vi "Read Total A-Scans.vi"(8 "error in (no error)":errorcluster, 11 "Scan in":refnum<class "Scan.lvclass">) -> (0 "error out":errorcluster, 2 "Total A-Scans":dbl, 3 "Scan out":refnum<class "Scan.lvclass">)   [LabVIEW 2017]
uses:
  Scan.lvclass
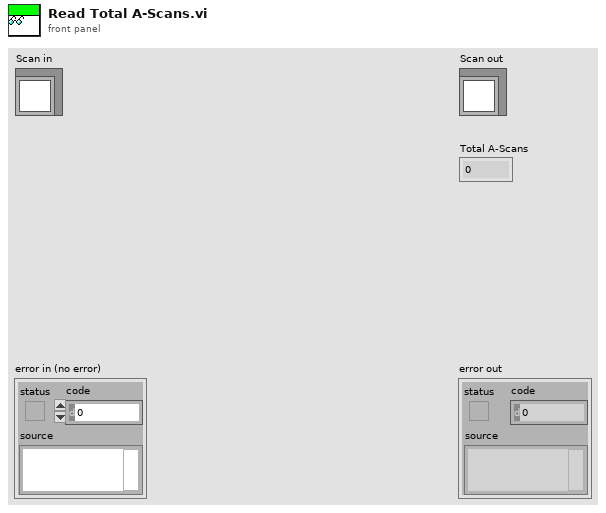
[diagram p1: front panel]
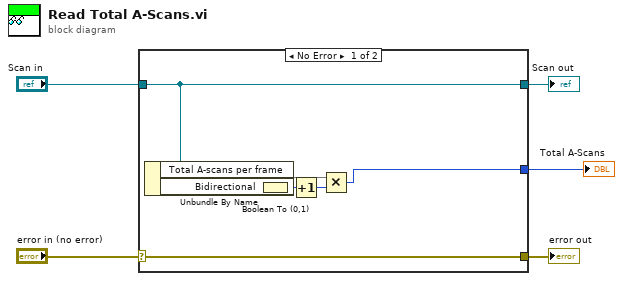
[diagram p0: block diagram]
diagram:
  n1 = case shown="No Error" "error in (no error)" {
    selector: "error in (no error)" -> [w12 w13]
    tunnel: [w12 w13] -> w4
    tunnel: [w11 w14] -> w2
    tunnel: "Scan in" -> [w11 w14]
    tunnel: [w6 _] -> w1
    frame No Error {
      n2 = Unbundle By Name(w11) -> ("Total A-scans per frame"=w7, "Bidirectional"=w10)
      n3 = Boolean To (0,1)(Boolean=w10) -> (0, 1=w9:i16)
      n4 = Increment(x=w9) -> (x+1=w8:i16)
      n5 = Multiply(x=w7, y=w8) -> (x*y=w6:i16)
    }
    frame Error {
    }
  }
  "error out" <- w4
  "Scan out" <- w2
  "Total A-Scans" <- w1
